vi "Cleanup.vi"(8 "error in (no error)":errorcluster, 11 "BuildManager in":refnum<class "BuildManager.lvclass">) -> (0 "error out":errorcluster, 3 "BuildManager out":refnum<class "BuildManager.lvclass">)   [LabVIEW 2020, in "SolutionBuilder.lvlib" / "BuildManager.lvclass"]
uses:
  BuildManager.lvclass
  BuildManager.lvclass/BuildManager.ctl
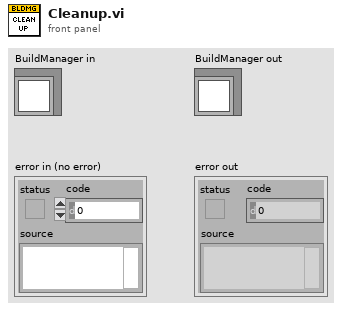
[diagram p1: front panel]
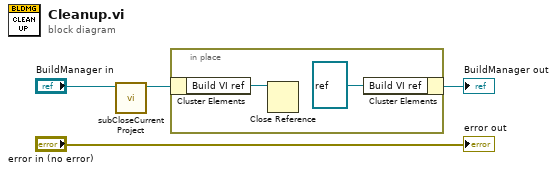
[diagram p0: block diagram]
diagram:
  n1 = call "subCloseCurrentProject.vi"("BuildManager in"="BuildManager in") -> ("BuildManager out"=w2:refnum<class "BuildManager.lvclass">)  [unwired: 9 in, 1 out]
  n2 = in-place {
    n3 = in-place-cluster #1(w2) -> ("Build VI ref"=w6:refnum<vi>)
    n4 = Close Reference(reference=w6) -> ()  [unwired: 1 in, 1 out]
    n5 = in-place-cluster #1("Build VI ref"=refnum<vi> refnum) -> (→"BuildManager out":refnum<class "BuildManager.lvclass">)
  }
  "error out" <- "error in (no error)"
